vi "Find Distance and Vector.vi"(10 "Point 2":cluster{"X":dbl, "Y":dbl}, 11 "Point 1":cluster{"X":dbl, "Y":dbl}) -> (2 "Distance":dbl, 3 "Unit Vector":cluster{"X":dbl, "Y":dbl})   [LabVIEW 2019, in "Tool Rectangle.lvclass"]
uses:
  Tool Rectangle.lvclass
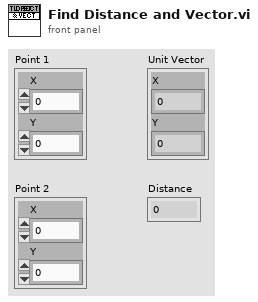
[diagram p1: front panel]
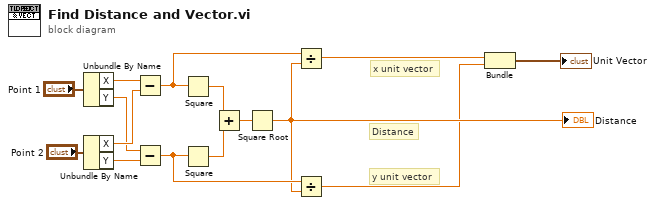
[diagram p0: block diagram]
diagram:
  # "Distance"
  # "y unit vector"
  # "x unit vector"
  n1 = Unbundle By Name("Point 1") -> ("X"=w15:dbl, "Y"=w12:dbl)
  n2 = Unbundle By Name("Point 2") -> ("X"=w14:dbl, "Y"=w13:dbl)
  n3 = Subtract(x=w15, y=w14) -> (x-y=w7:dbl)
  n4 = Subtract(x=w12, y=w13) -> (x-y=w8:dbl)
  n5 = Square(x=w7) -> (x^2=w11:dbl)
  n6 = Square(x=w8) -> (x^2=w10:dbl)
  n7 = Add(x=w11, y=w10) -> (x+y=w9:dbl)
  n8 = Square Root(x=w9) -> (sqrt(x)=w6:dbl)
  "Distance" <- w6
  n9 = Divide(x=w7, y=w6) -> (x/y=w2:dbl)
  n10 = Divide(x=w8, y=w6) -> (x/y=w1:dbl)
  n11 = Bundle(w2, w1) -> (→"Unit Vector":cluster{dbl, dbl})  [unwired: 1 in]
